vi "Run Test.vi"(8 "error in (no error)":errorcluster, 11 "Test Template in":refnum<class "Enable String Loads.lvclass">) -> (0 "error out":errorcluster, 1 "Positions":i32[](array[numeric]), 2 "Tests Passed":bool[](array[boolean]), 3 "Test Template out":refnum<class "Enable String Loads.lvclass">, 5 "Fail Codes":string[](array[string]))   [LabVIEW 2015, in "Enable String Loads.lvclass"]
uses:
  Enable String Loads.lvclass
  Classes/Application/Class/Application.lvclass
  Test Class/Test Class.lvclass
  Driver Test/Driver Test.lvclass
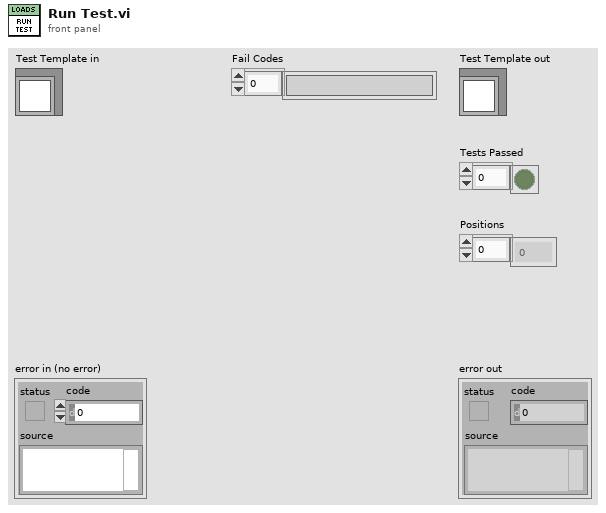
[diagram p1: front panel]
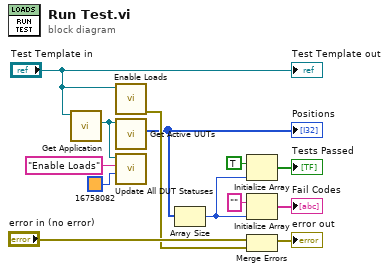
[diagram p0: block diagram]
diagram:
  n1 = call "Get Application.vi"("Test Class in"="Test Template in") -> ("Application.lvlib:Application.lvclass"=w9:refnum<class "Application.lvclass">)  [unwired: 9 in, 1 out]
  n2 = call "Enable Loads.vi"("Driver Test in"="Test Template in") -> ("error out"=w7:errorcluster)  [unwired: 10 in]
  n3 = call "Get Active UUTs.vi"("Application in"=w9) -> ("Active Positions"=w6:u32[])  [unwired: 8 in, 2 out]
  "Positions" <- w6
  n4 = call "Update All DUT Statuses.vi"("BG Color"=u32 16758082, "Message ('')"="Enable Loads", "Application in"=w9) -> ()  [unwired: 7 in, 2 out]
  n5 = Array Size(array=w6) -> (size(s)=w5:i32)
  n6 = Initialize Array(TRUE, w5) -> (→"Tests Passed":bool[])
  n7 = Initialize Array("", w5) -> (→"Fail Codes":string[])
  n8 = Merge Errors("error in (no error)", w7) -> (→"error out":errorcluster)
  "Test Template out" <- "Test Template in"
